vi "Save Word Report to File.vi"(0 "report in":refnum<class "NI_report.lvclass">, 5 "report file path (*.docx)":path, 11 "error in (no error)":errorcluster) -> (4 "report out":refnum<class "NI_report.lvclass">, 15 "error out":errorcluster)   [LabVIEW 2018, in "WordReportGeneration.lvlib" / "Word_Report.lvclass"]
uses:
  Word_Report.lvclass
  <vilib>/Utility/NIReport.llb/NI_report.lvclass
  <vilib>/Utility/NIReport.llb/Word/NI_Word.lvclass
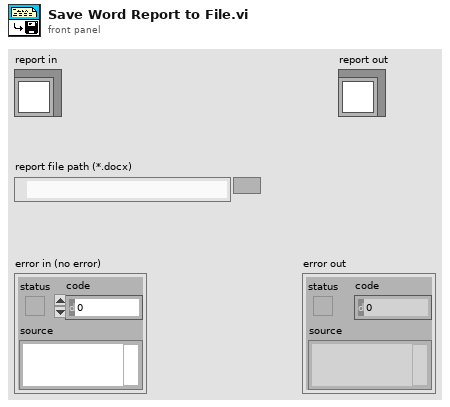
[diagram p1: front panel]
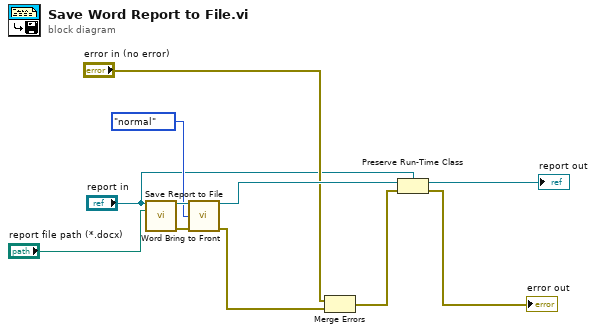
[diagram p0: block diagram]
diagram:
  n1 = call-dynamic "Save Report to File.vi"("report in"="report in", "report file path"="report file path (*.docx)") -> ("report out"=w11:refnum<class "NI_report.lvclass">, "error out"=w6:errorcluster)  [unwired: 12 in]
  n2 = call <vilib>:"Word Bring to Front.vi"("report in"=w11, "window state (maximized)"=enum16{"maximized", "minimized", "normal"}."normal", "error in (no error)"=w6) -> ("report out"=w9:refnum<class "NI_report.lvclass">, "error out"=w1:errorcluster)  [unwired: 11 in]
  n3 = Merge Errors("error in (no error)", w1) -> (w3:errorcluster)
  n4 = Preserve Run-Time Class(object in=w9, error in=w3, 2:"report in") -> (object out=→"report out":refnum<class "NI_report.lvclass">, error out=→"error out":errorcluster)
